vi "GFITS_Readfile2fits.vi"(10 "def_timing":string="after", 11 "file":path) -> (0 "number of before keywords":i32, 1 "before Keywords":string[][](array[string]), 2 "number of after keywords":i32, 3 "after Keywords":string[][](array[string]), 4 "all keys":string[][](array[string]), 6 "number of total keywords":i32)   [LabVIEW 2016]
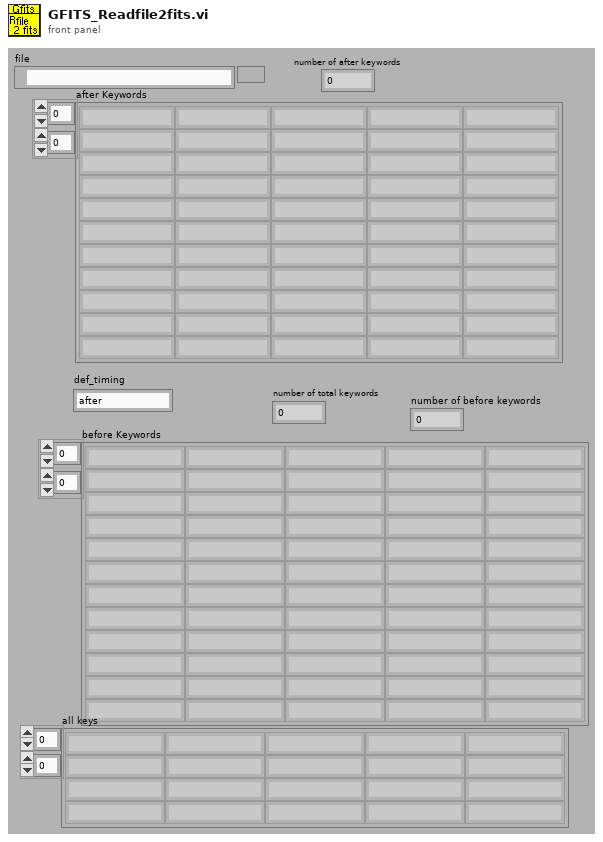
[diagram p1: front panel]
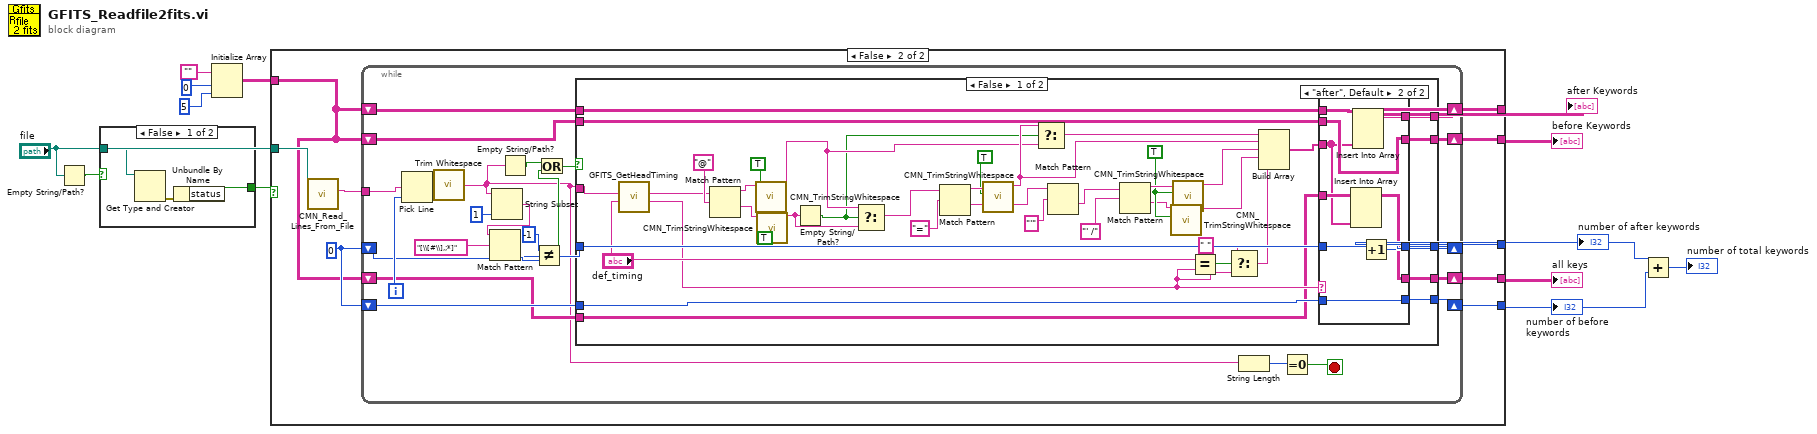
[diagram p0: block diagram]
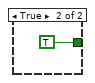
[diagram p2: hidden frame]
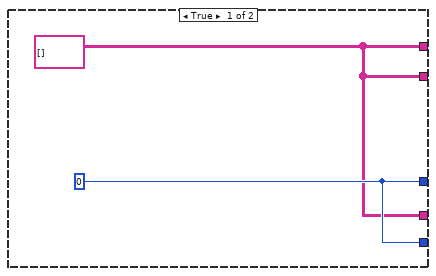
[diagram p3: hidden frame]
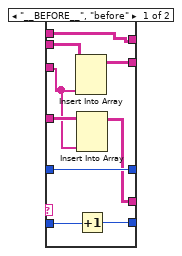
[diagram p4: hidden frame]
diagram:
  n1 = Empty String/Path?(string/path="file") -> (empty?=w7:bool)
  n2 = case shown="False" w7 {
    tunnel: "file" -> [w15 _]
    tunnel: [w14 TRUE ("status")] -> w9
    frame False {
      n3 = Get Type and Creator(7:w15) -> (0:w16:errorcluster)  [unwired: 1 in, 3 out]
      n4 = Unbundle By Name(w16) -> ("status"=w14:bool)
    }
    frame True {
    }
  }
  n5 = Initialize Array("", 0, 5) -> (w10:string[][])
  n6 = case shown="False" w9 {
    tunnel: "file" -> [_ w26]
    tunnel: [w19 w25] -> w3
    tunnel: [w18 w27] -> w6
    tunnel: w10 -> [_ w21]
    tunnel: [w18 w23] -> w5
    tunnel: [w19 w22] -> w2
    tunnel: [w18 w20] -> w4
    frame True {
      w18 = string[][] []
      w19 = 0
    }
    frame False {
      w24 = 0
      n7 = call "CMN_Read_Lines_From_File.vi"("file path"=w26) -> ("line string"=w28:string)  [unwired: 1 in, 7 out]
      n8 = while {
        shift-left: w24 -> [w44]
        shift-right: [w46] -> w25
        shift-left: w21 -> [w50]
        shift-right: [w49] -> w27
        tunnel: w28 -> [w31]
        shift-right: [w40] -> w23
        shift-left: w21 -> [w39]
        shift-right: [w38] -> w22
        shift-left: w24 -> [w37]
        shift-right: [w35] -> w20
        shift-left: w21 -> [w36]
        i -> [w45]
        stop <- w51 stop-if-true
        n9 = Pick Line(multi-line string=w31, line index=w45) -> (output string=w34:string)  [unwired: 1 out]
        n10 = call <vilib>:"Trim Whitespace.vi"("string"=w34) -> ("trimmed string"=w30:string)  [unwired: 1 in]
        n11 = String Subset(string=w30, length (rest)=1 ("length (rest)")) -> (substring=w32:string)  [unwired: 1 out]
        n12 = Match Pattern(string=w32, regular expression="[\\[#\\],;*]") -> (offset past match=w48:i32)  [unwired: 4 out]
        n13 = Empty String/Path?(string/path=w30) -> (empty?=w43:bool)
        n14 = Not Equal?(x=-1, y=w48) -> (x != y?=w42:bool)
        n15 = Or(x=w43, y=w42) -> (x .or. y?=w41:bool)
        n16 = case shown="False" w41 {
          tunnel: w44 -> [w62 w115]
          tunnel: w50 -> [w80 w116]
          tunnel: [w79 w116] -> w49
          tunnel: [w65 w115] -> w46
          tunnel: w30 -> [w67 _]
          tunnel: [w64 w114] -> w40
          tunnel: w39 -> [w63 w114]
          tunnel: [w61 w113] -> w38
          tunnel: w37 -> [w60 w113]
          tunnel: w36 -> [w54 w112]
          tunnel: [w53 w112] -> w35
          frame False {
            w85 = TRUE ("Both Ends?(F)")
            n17 = call "GFITS_GetHeadTiming.vi"("def_timing"="def_timing", "line In"=w67) -> ("head_tim"=w57:string, "line out"=w66:string)  [unwired: 8 out]
            n18 = Match Pattern(string=w66, regular expression="@") -> (before substring=w74:string, after substring=w76:string)  [unwired: 3 out]
            n19 = call "CMN_TrimStringWhitespace.vi"("Both Ends?(T)"=TRUE ("Both Ends?(F)"), "string"=w74) -> ("trimmed string"=w70:string)  [unwired: 8 out]
            n20 = call "CMN_TrimStringWhitespace.vi"("Both Ends?(T)"=TRUE ("Both Ends?(F)"), "string"=w76) -> ("trimmed string"=w73:string)  [unwired: 8 out]
            n21 = Empty String/Path?(string/path=w73) -> (empty?=w68:bool)
            n22 = Select(t=w70, s=w68, f=w73) -> (s? t:f=w72:string)
            n23 = Match Pattern(string=w72, regular expression="=") -> (before substring=w92:string, after substring=w91:string)  [unwired: 3 out]
            n24 = call "CMN_TrimStringWhitespace.vi"("Both Ends?(T)"=TRUE ("Both Ends?(F)"), "string"=w92) -> ("trimmed string"=w71:string)  [unwired: 8 out]
            n25 = Select(t=w71, s=w68, f=w70) -> (s? t:f=w69:string)
            n26 = Match Pattern(string=w91, regular expression="'") -> (after substring=w89:string)  [unwired: 4 out]
            n27 = Match Pattern(string=w89, regular expression="' /") -> (before substring=w87:string, after substring=w84:string)  [unwired: 3 out]
            n28 = call "CMN_TrimStringWhitespace.vi"("Both Ends?(T)"=w85, "string"=w84) -> ("trimmed string"=w82:string)  [unwired: 8 out]
            n29 = call "CMN_TrimStringWhitespace.vi"("Both Ends?(T)"=w85, "string"=w87) -> ("trimmed string"=w83:string)  [unwired: 8 out]
            n30 = Equal?(x="def_timing", y=w57) -> (x = y?=w58:bool)
            n31 = Select(t=" ", s=w58, f=w57) -> (s? t:f=w55:string)
            n32 = Build Array(w69, w71, w83, w82, w55) -> (w81:string[])
            n33 = case shown="\"after\", Default" w57 {
              tunnel: w81 -> [w95 w103]
              tunnel: w80 -> [w102 w111]
              tunnel: [w102 w110] -> w79
              tunnel: w62 -> [w99 w109]
              tunnel: [w99 w108] -> w65
              tunnel: [w101 w106] -> w64
              tunnel: w63 -> [w100 w106]
              tunnel: [w98 w107] -> w61
              tunnel: w60 -> [w97 w107]
              tunnel: w54 -> [w96 w105]
              tunnel: [w94 w104] -> w53
              frame "__BEFORE__", "before" {
                n34 = Insert Into Array(array=w100, new element=w95) -> (w101:string[][])  [unwired: 2 in]
                n35 = Insert Into Array(array=w96, new element=w95) -> (w94:string[][])  [unwired: 2 in]
                n36 = Increment(x=w97) -> (x+1=w98:i32)
              }
              frame "after", Default {
                n37 = Insert Into Array(array=w105, new element=w103) -> (w104:string[][])  [unwired: 2 in]
                n38 = Insert Into Array(array=w111, new element=w103) -> (w110:string[][])  [unwired: 2 in]
                n39 = Increment(x=w109) -> (x+1=w108:i32)
              }
            }
          }
          frame True {
          }
        }
        n40 = String Length(string=w30) -> (length=w52:i32)
        n41 = Equal To 0?(x=w52) -> (x = 0?=w51:bool)
      }
    }
  }
  "number of after keywords" <- w3
  "after Keywords" <- w6
  "before Keywords" <- w5
  "number of before keywords" <- w2
  "all keys" <- w4
  n42 = Add(x=w3, y=w2) -> (x+y=→"number of total keywords":i32)
